vi "ZeroMyOrigin.vi"(5 "error in (no error)":errorcluster) -> (19 "error out":errorcluster)   [LabVIEW 2023]
panel:
  out "Name of calling VI":string
  # "Adjust the VI's front panel to put origin at 0, 0"
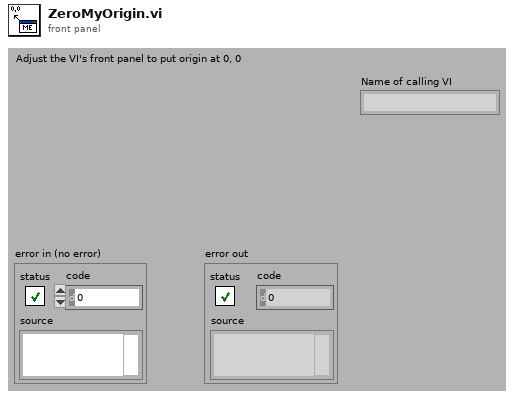
[diagram p1: front panel]
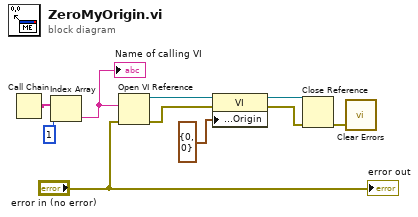
[diagram p0: block diagram]
diagram:
  n1 = Call Chain() -> (call chain=w10:string[])
  n2 = Index Array(array=w10, index=1) -> (element=w9:string)
  "Name of calling VI" <- w9
  n3 = Open VI Reference(vi path=w9, error in (no error)="error in (no error)") -> (vi reference=w7:refnum<vi>, error out=w5:errorcluster)  [unwired: 4 in]
  n4 = property class="VI"(reference=w7, error in=w5, "Front Panel Window:Origin"=cluster{"Horizontal":i16, "Vertical":i16} {"Horizontal"=0, "Vertical"=0}) -> (reference out=w3:refnum<vi>, error out=w4:errorcluster)
  n5 = Close Reference(reference=w3, error in (no error)=w4) -> (error out=w2:errorcluster)
  n6 = call <vilib>:"Clear Errors.vi"("error in (no error)"=w2) -> ()  [unwired: 5 in, 2 out]
  "error out" <- "error in (no error)"
